vi "testTime.vi"() -> ()   [LabVIEW 2019, in "TestResultTest.lvlib"]
uses:
  TestResultTest.lvlib
  TestResult/TestResult.lvclass
  Support/TestCaseMock/TestCaseMock.lvclass
  C:/Users/de200256/Code/LVUnit/TestCase/TestCase/TestCase.lvclass
  e093cbbb-51c9-49d7-a546-16803894d9b6.vi
  Constraint/IsEqual/IsEqual.lvclass
  C:/Users/de200256/Code/LVUnit/Constraint/Constraint/Constraint.lvclass
  Constraint/IsEqual/Create.vi
  Constraint/LogicalNot/LogicalNot.lvclass
  Constraint/UnaryOperator/UnaryOperator.lvclass
  C:/Users/de200256/Code/LVUnit/Test/Test.lvclass
panel:
  out "error out":errorcluster
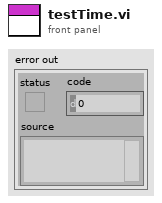
[diagram p1: front panel]
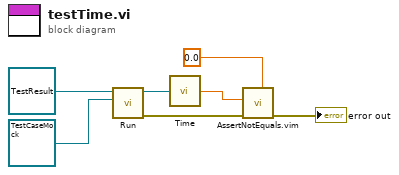
[diagram p0: block diagram]
diagram:
  n1 = call-dynamic "Run.vi"("TestCase"=refnum<class "TestCaseMock.lvclass"> refnum ("TestCase.lvclass"), "TestResult in"=refnum<class "TestResult.lvclass"> refnum ("TestResult.lvclass")) -> ("error out"=w5:errorcluster, "TestResult out"=w6:refnum<class "TestResult.lvclass">)  [unwired: 7 in, 1 out]
  n2 = call "Time.vi"("TestResult In"=w6) -> ("Time"=w2:dbl)
  n3 = call "AssertNotEquals.vim"("Expected"=0.0, "error in (no error)"=w5, "Actual"=w2) -> ("error out"=→"error out":errorcluster)  [unwired: 8 in]
